vi "Get Robot Config.vi"() -> (1 "LL Constants":T1, 2 "Shooter Table":dbl[][](array[numeric]))   [LabVIEW 2023]
uses:
  <vilib>/Rock Robotics/Network Tables/NT Read Number.vi
panel:
  in  "2468 Competition":dbl[][](array[numeric])=[[4600.0, 700.0, 4600.0, 4000.0, 0.0, 700.0, 3000.0], [4600.0, 1600.0, 4600.0, 4000.0, 0.0, 700.0, 2500.0], [3.0, 7.5, 6.5, 7.5, 0.0, 0.0, 7.0]]
  in  "2468 Competition LL Constants":T1={"LL Angle"=18.0, "LL Height"=21.0, "Bumper Width"=17.0}
  in  "2468 Practice":dbl[][](array[numeric])=[[5500.0, 1000.0, 6000.0, 0.0, 0.0, 700.0, 2300.0], [4000.0, 1900.0, 5000.0, 0.0, 0.0, 700.0, 2000.0], [0.0, 0.0, 0.0, 0.0, 0.0, 0.0, 10.0]]
  in  "2468 Practice LL Constants":T1
  # "Speaker, Amp, Subwoofer, Stage, Zero, Idle, Trap"
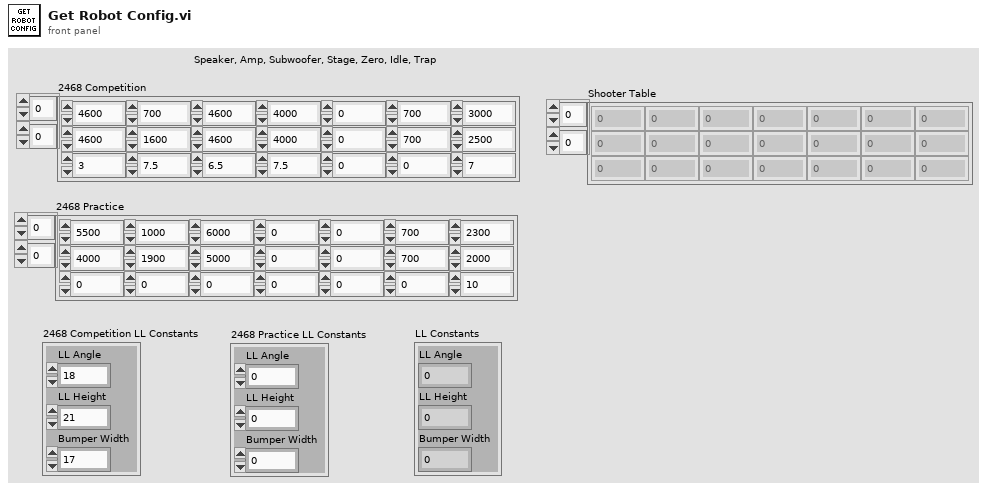
[diagram p1: front panel]
types:
  T1 = cluster{"LL Angle":dbl, "LL Height":dbl, "Bumper Width":dbl}
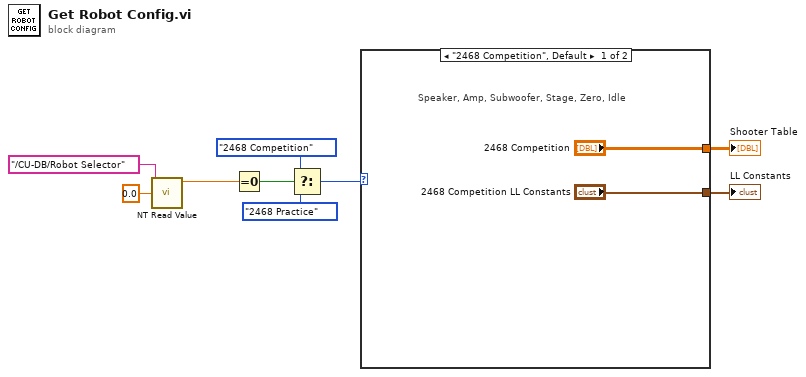
[diagram p0: block diagram]
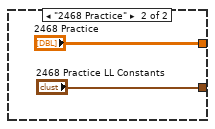
[diagram p2: hidden frame]
diagram:
  n1 = call-poly <vilib>:"NT Read Value.vi"("default value"=0.0, "name"="/CU-DB/Robot Selector") -> ("value"=w8:dbl)  [unwired: 7 in, 2 out]
  n2 = Equal To 0?(x=w8) -> (x = 0?=w7:bool)
  n3 = Select(t=enum16{"2468 Competition", "2468 Practice"}."2468 Competition", s=w7, f=enum16{"2468 Competition", "2468 Practice"}."2468 Practice") -> (s? t:f=w2:enum16{"2468 Competition", "2468 Practice"})
  n4 = case shown="\"2468 Competition\", Default" w2 {
    tunnel: ["2468 Competition" "2468 Practice"] -> w3
    tunnel: ["2468 Competition LL Constants" "2468 Practice LL Constants"] -> w1
    frame "2468 Competition", Default {
      # "Speaker, Amp, Subwoofer, Stage, Zero, Idle"
    }
    frame "2468 Practice" {
    }
  }
  "Shooter Table" <- w3
  "LL Constants" <- w1
